vi "Create Evaluations.vi"(8 "error in (no error)":errorcluster, 11 "IEvaluation in":refnum<class "PAE.lvclass">) -> (0 "error out":errorcluster, 2 "Evaluations Out":T1[](array[typedef]) {"Low Limit" format="%#_13g"; "SI Scaling" items=["femto"=-15, "pico"=-12, "nano"=-9, "micro"=-6, "milli"=-3, "percent"=-2, ""=0, "kilo"=3, "mega"=6, "giga"=9, "tera"=12]}, 3 "IEvaluation out":refnum<class "PAE.lvclass">)   [LabVIEW 2016, in "SeqAuto Evaluations.lvlib" / "PAE.lvclass"]
uses:
  PAE.lvclass
  C:/Sequence Automation/Plugins/SeqAuto IEvaluation.lvlibp/SeqAuto IEvaluation.lvclass
  Plugins/TestStand API Tools (TSAT).lvlibp/Evaluation Actions/Includes/Controls/TSAT Evaluation.ctl
  Plugins/TestStand API Tools (TSAT).lvlibp/Evaluation Actions/Includes/Controls/TSAT Eval SI Unit Scaling.ctl
  Plugins/TestStand API Tools (TSAT).lvlibp/Evaluation Actions/Includes/Controls/TSAT Evaluation Type.ctl
  PAE.lvclass/PAE.ctl
  Read SA Pin.vi
  Plugins/SeqAuto IEvaluation.lvlibp/Read Measurement Name.vi
  Plugins/TestStand API Tools (TSAT).lvlibp/Evaluation Actions/TSAT Evaluation Actions.lvlib
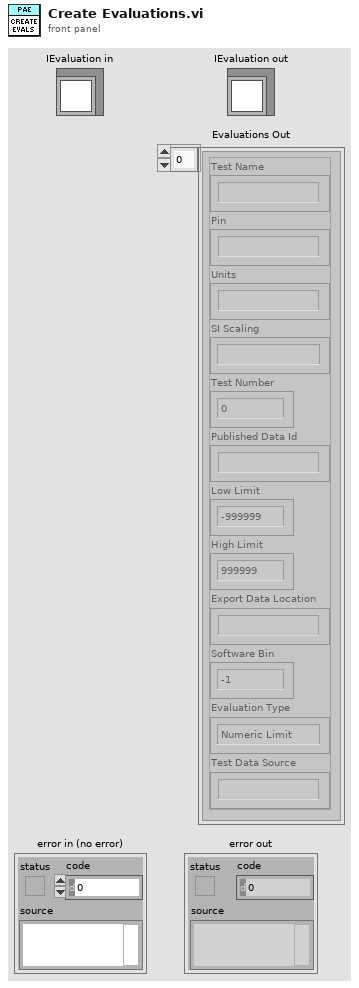
[diagram p1: front panel]
types:
  T1 = typedef "TestStand API Tools (TSAT).lvlibp/TSAT Evaluation Actions.lvlib/TSAT Evaluation.ctl" = cluster{"Test Name":string, "Pin":string, "Units":string, "SI Scaling":T2, "Test Number":i32, "Published Data Id":string, "Low Limit":dbl, "High Limit":dbl, "Export Data Location":string, "Software Bin":i64, "Evaluation Type":T3, "Test Data Source":string}
  T2 = typedef "TestStand API Tools (TSAT).lvlibp/TSAT Evaluation Actions.lvlib/TSAT Eval SI Unit Scaling.ctl" = i16
  T3 = typedef "TestStand API Tools (TSAT).lvlibp/TSAT Evaluation Actions.lvlib/TSAT Evaluation Type.ctl" = enum16{"Numeric Limit", "Pass/Fail", "None"}
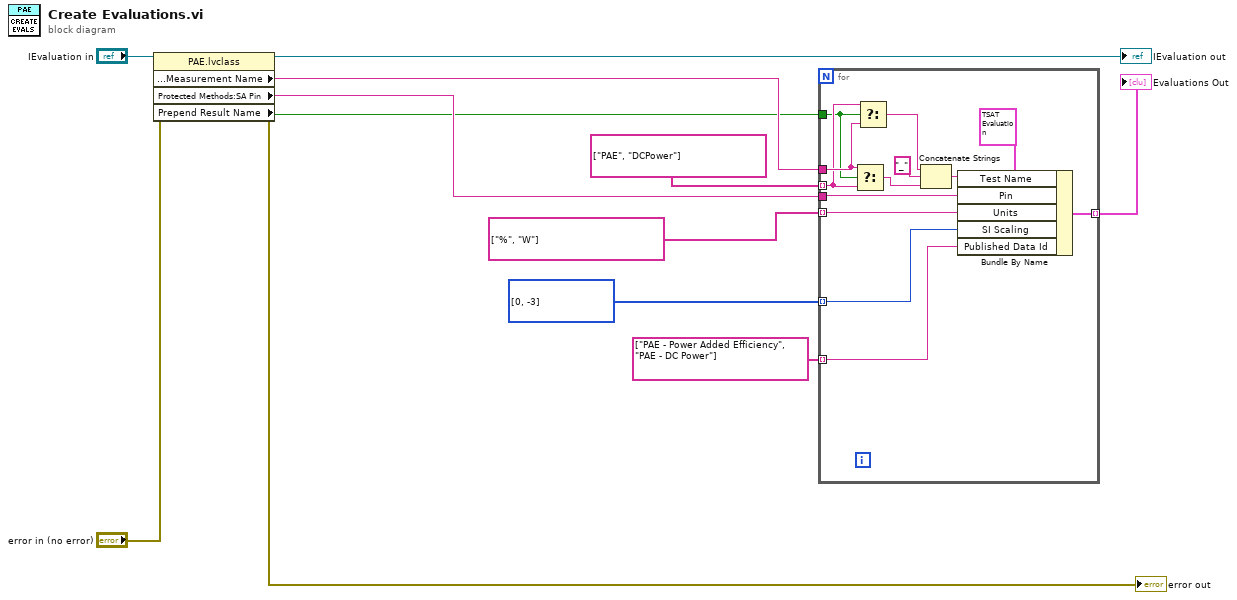
[diagram p0: block diagram]
diagram:
  w10 = T2[] [0, -3] items=["femto"=-15, "pico"=-12, "nano"=-9, "micro"=-6, "milli"=-3, "percent"=-2, ""=0, "kilo"=3, "mega"=6, "giga"=9, "tera"=12]
  n1 = property class="PAE.lvclass"(reference="IEvaluation in", error in="error in (no error)") -> (reference out=→"IEvaluation out":refnum<class "PAE.lvclass">, error out=→"error out":errorcluster, "Protected Methods:Measurement Name"=w4:string, "Protected Methods:SA Pin"=w3:string, "Prepend Result Name"=w1:bool)
  n2 = for {
    tunnel: [w24] -> w7 mode=indexing
    tunnel: w4 -> [w16]
    tunnel: string[] ["PAE", "DCPower"] -> [w14] mode=indexing
    tunnel: w10 -> [w22] mode=indexing
    tunnel: string[] ["%", "W"] -> [w21] mode=indexing
    tunnel: string[] ["PAE - Power Added Efficiency", "PAE - DC Power"] -> [w20] mode=indexing
    tunnel: w3 -> [w18]
    tunnel: w1 -> [w13]
    n3 = Select(t=w16, s=w13, f=w14) -> (s? t:f=w15:string)
    n4 = Select(t=w14, s=w13, f=w16) -> (s? t:f=w17:string)
    n5 = Concatenate Strings(w17, "_" ("string"), w15) -> (w23:string)
    n6 = Bundle By Name(cluster=T1 {"Test Name"="", "Pin"="", "Units"="", "SI Scaling"=0, "Test Number"=0, "Published Data Id"="", "Low Limit"=-999999.0, "High Limit"=999999.0, "Export Data Location"="", "Software Bin"=-1, "Evaluation Type"=enum."Numeric Limit", "Test Data Source"=""} ("Evaluation"), "Test Name"=w23, "Pin"=w18, "Units"=w21, "SI Scaling"=w22, "Published Data Id"=w20) -> (w24:T1)
  }
  "Evaluations Out" <- w7
